vi "Example Subscriber.vi"() -> ()   [LabVIEW 2021]
uses:
  TCP_Streamer_Subscriber/Typedef/State.ctl
  TCP_Streamer_Subscriber/Typedef/Configuration.ctl
  TCP_Streamer_Subscriber/TCP_Streamer_Subscriber.lvclass/TCP_Streamer_Subscriber.ctl
  TCP_Streamer_Subscriber/TCP_Streamer_Subscriber.lvclass
panel:
  out "Timeout":bool
  in  "Configuration":T1={"Remote Address"="localhost", "Remote Port"=0, "Local Port"=0}
  out "State":T2
  out "Fault":bool
  in  "stop":bool
  out "error out":errorcluster
  out "data out":string
  in  "delay (ms)":u32=50
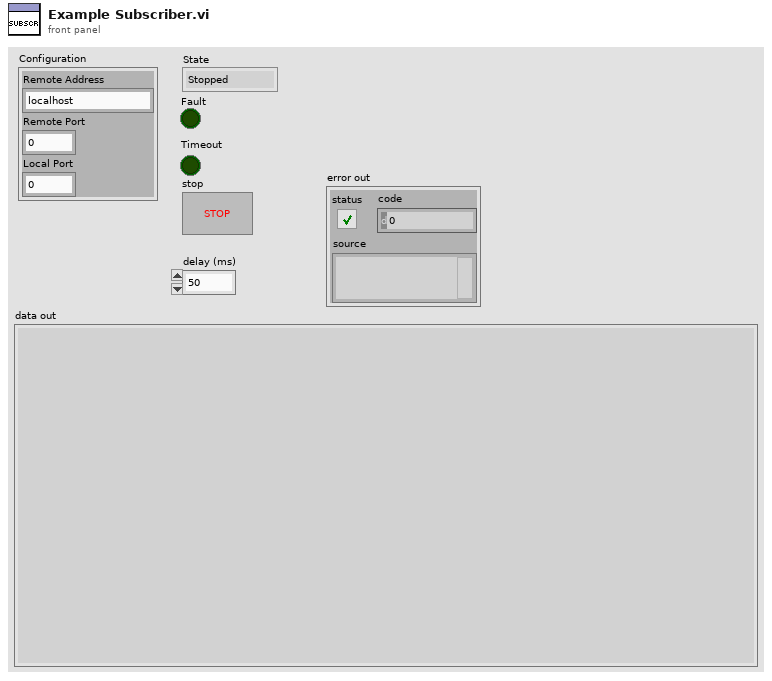
[diagram p1: front panel]
types:
  T1 = typedef "TCP_Streamer_Subscriber.lvclass/Configuration.ctl" = cluster{"Remote Address":string, "Remote Port":u16, "Local Port":u16}
  T2 = typedef "TCP_Streamer_Subscriber.lvclass/State.ctl" = enum16{"Stopped", "Connecting", "Receiving"}
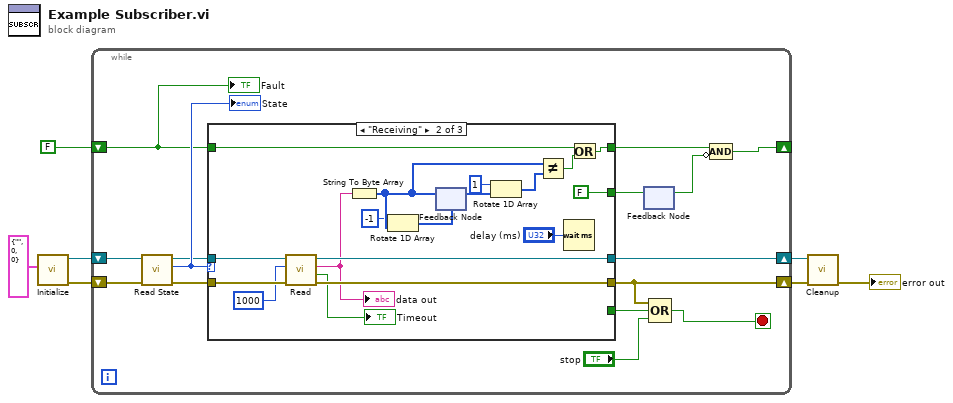
[diagram p0: block diagram]
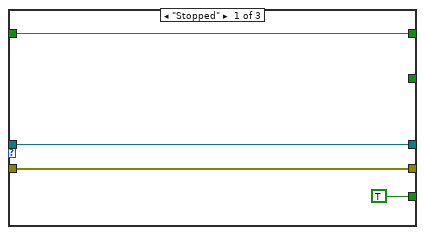
[diagram p2: hidden frame]
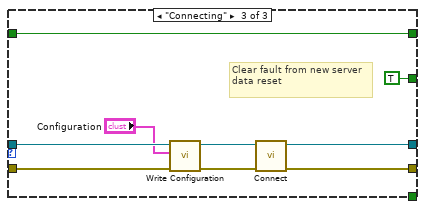
[diagram p3: hidden frame]
diagram:
  n1 = call "Initialize.vi"("Configuration"=T1 {"Remote Address"="", "Remote Port"=0, "Local Port"=0}) -> ("error out"=w6:errorcluster, "TCP_Streamer_Subscriber out"=w7:refnum<class "TCP_Streamer_Subscriber.lvclass">)  [unwired: 9 in]
  n2 = while {
    shift-right: [w17] -> w5
    shift-left: w7 -> [w22]
    shift-right: [w15] -> w4
    shift-left: w6 -> [w21]
    shift-right: [w10] -> _
    shift-left: FALSE -> [w16]
    stop <- w14 stop-if-true
    n3 = call "Read State.vi"("error in (no error)"=w21, "TCP_Streamer_Subscriber in"=w22) -> ("error out"=w18:errorcluster, "State"=w20:T2, "TCP_Streamer_Subscriber out"=w19:refnum<class "TCP_Streamer_Subscriber.lvclass">)  [unwired: 7 in]
    "State" <- w20
    n4 = case shown="\"Receiving\"" w20 {
      tunnel: w19 -> [w26 w44 w50]
      tunnel: w18 -> [w25 w43 w49]
      tunnel: [w26 w41 w53] -> w17
      tunnel: [w25 w42 w52] -> w15
      tunnel: w16 -> [w24 w31 w51]
      tunnel: [w24 w29 w51] -> w11
      tunnel: [TRUE _ _] -> w12
      tunnel: [_ FALSE TRUE] -> w9
      frame "Stopped" {
      }
      frame "Receiving" {
        n5 = call "Read.vi"("error in (no error)"=w43, "bytes to read"=1000, "TCP_Streamer_Subscriber in"=w44) -> ("error out"=w42:errorcluster, "Timeout"=→"Timeout":bool, "data out"=w32:string, "TCP_Streamer_Subscriber out"=w41:refnum<class "TCP_Streamer_Subscriber.lvclass">)  [unwired: 5 in]
        "data out" <- w32
        n6 = String To Byte Array(string=w32) -> (unsigned byte array=w38:u8[])
        n7 = Rotate 1D Array(1:w38, 2:-1 ("n")) -> (0:w36:u8[])
        n8 = feedback #1(w36) -> (w33:u8[])
        n9 = feedback-in #1(w38) -> ()
        n10 = Rotate 1D Array(1:w33, 2:1 ("n")) -> (0:w37:u8[])
        n11 = Not Equal?(x=w38, y=w37) -> (x != y?=w30:bool)
        n12 = Wait (ms)(milliseconds to wait="delay (ms)") -> ()  [unwired: 1 out]
        n13 = Or(x=w31, y=w30) -> (x .or. y?=w29:bool)
      }
      frame "Connecting" {
        # "Clear fault from new server data reset"
        n14 = call "Write Configuration.vi"("error in (no error)"=w49, "Configuration"="Configuration", "TCP_Streamer_Subscriber in"=w50) -> ("error out"=w47:errorcluster, "TCP_Streamer_Subscriber out"=w48:refnum<class "TCP_Streamer_Subscriber.lvclass">)  [unwired: 7 in]
        n15 = call "Connect.vi"("error in (no error)"=w47, "TCP_Streamer_Subscriber in"=w48) -> ("error out"=w52:errorcluster, "TCP_Streamer_Subscriber out"=w53:refnum<class "TCP_Streamer_Subscriber.lvclass">)  [unwired: 8 in]
      }
    }
    n16 = feedback-in #2(w9) -> ()
    n17 = feedback #2() -> (w8:bool)  [unwired: 1 in]
    n18 = Compound Arithmetic op=OR(w15, w12, "stop") -> (w14:bool)
    n19 = Compound Arithmetic op=AND(w11, invert w8) -> (w10:bool)
    "Fault" <- w16
  }
  n20 = call "Cleanup.vi"("error in (no error)"=w4, "TCP_Streamer_Subscriber in"=w5) -> ("error out"=→"error out":errorcluster)  [unwired: 8 in, 1 out]
